vi "piezo-cluster.vi"(2 "cluster carte entree":T3, 3 "cluster carte data":T1) -> (0 "cluster carte sortie":T2, 1 "voltage (V)":dbl)   [LabVIEW 2019]
uses:
  <vilib>/DAQmx/write.llb/DAQmx Write (Analog DBL 1Chan 1Samp).vi
  <vilib>/DAQmx/miscellaneous.llb/DAQmx Fill In Error Info.vi
panel:
  # "SORTIES"
  # "ENTREES"
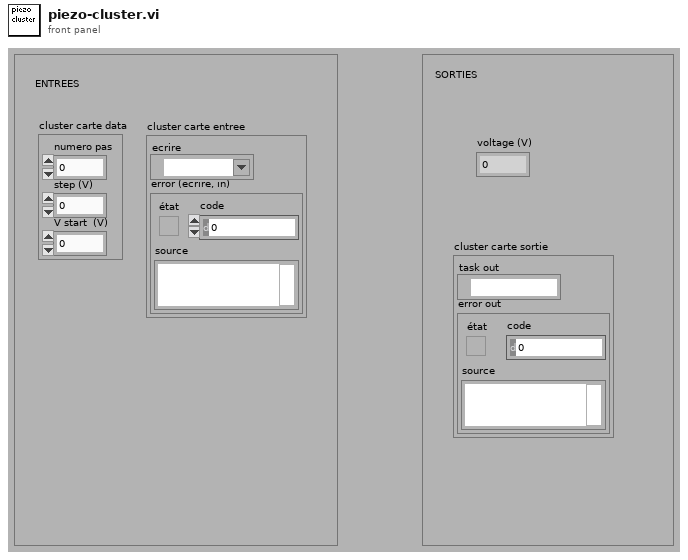
[diagram p1: front panel]
types:
  T1 = cluster{"numero pas":i32, "step (V)":dbl, "V start  (V)":dbl}
  T2 = cluster{"task out":refnum<k21>, "error out":errorcluster}
  T3 = cluster{"ecrire":refnum<k21>, "error (ecrire, in)":errorcluster}
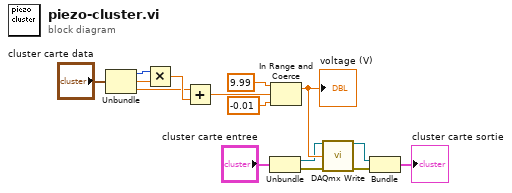
[diagram p0: block diagram]
diagram:
  n1 = Unbundle("cluster carte data") -> ("numero pas"=w3:i32, "step (V)"=w2:dbl, "V start  (V)"=w1:dbl)
  n2 = Multiply(x=w3, y=w2) -> (x*y=w12:dbl)
  n3 = Add(x=w1, y=w12) -> (x+y=w11:dbl)
  n4 = Unbundle("cluster carte entree") -> ("ecrire"=w9:refnum<k21>, "error (ecrire, in)"=w8:errorcluster)
  n5 = In Range and Coerce(upper limit=9.99 ("limite haute"), x=w11, lower limit=-0.01 ("limite basse")) -> (coerced(x)=w15:dbl)  [unwired: 1 out]
  "voltage (V)" <- w15
  n6 = call-poly <vilib>:"DAQmx Write.vi"("task/channels in"=w9, "data"=w15, "error in"=w8) -> ("task out"=w7:refnum<k21>, "error out"=w6:errorcluster)  [unwired: 1 in, 10 out]
  n7 = Bundle("task out"=w7, "error out"=w6) -> (→"cluster carte sortie":T2)  [unwired: 1 out]
